vi "SequenceStructures.vi"() -> ()   [LabVIEW 2025]
uses:
  <vilib>/numeric/Random Number (Range) DBL.vi
panel:
  in  "Path 4":path
  out "Waveform Chart 4":dynamicdata(graph)
  in  "lower limit 2":dbl
  in  "upper limit 2":dbl
  in  "?":bool
  in  "write to file 2":bool
  in  "Path 3":path
  out "temperature 2":dbl
  out "Waveform Chart 3":dbl(graph)
  out "Waveform Chart 2":dynamicdata(graph)
  in  "Path 2":path
  in  "lower limit":dbl
  in  "upper limit":dbl
  in  "?":bool
  in  "write to file":bool
  in  "Path":path
  out "temperature":dbl
  out "Waveform Chart":dbl(graph)
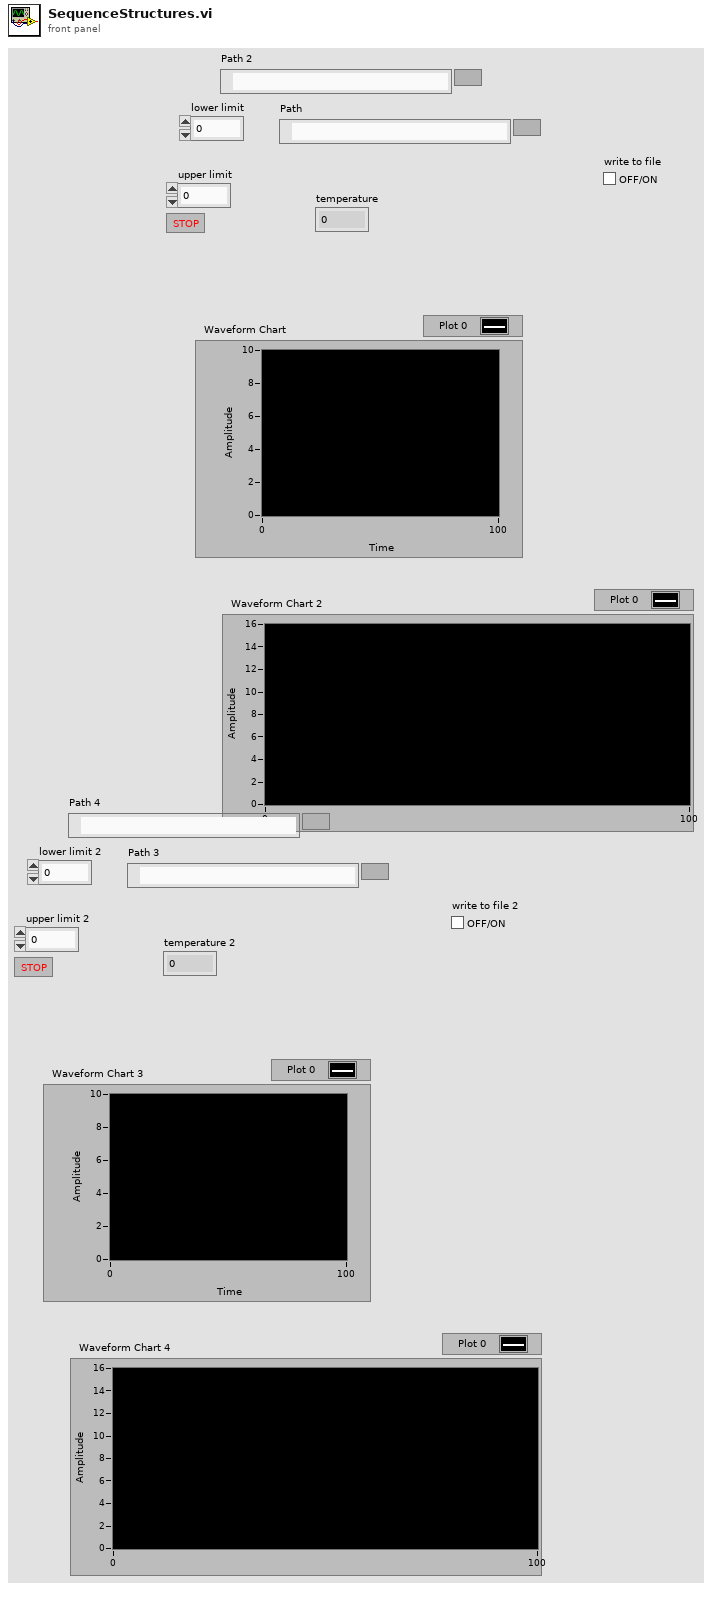
[diagram p1: front panel]
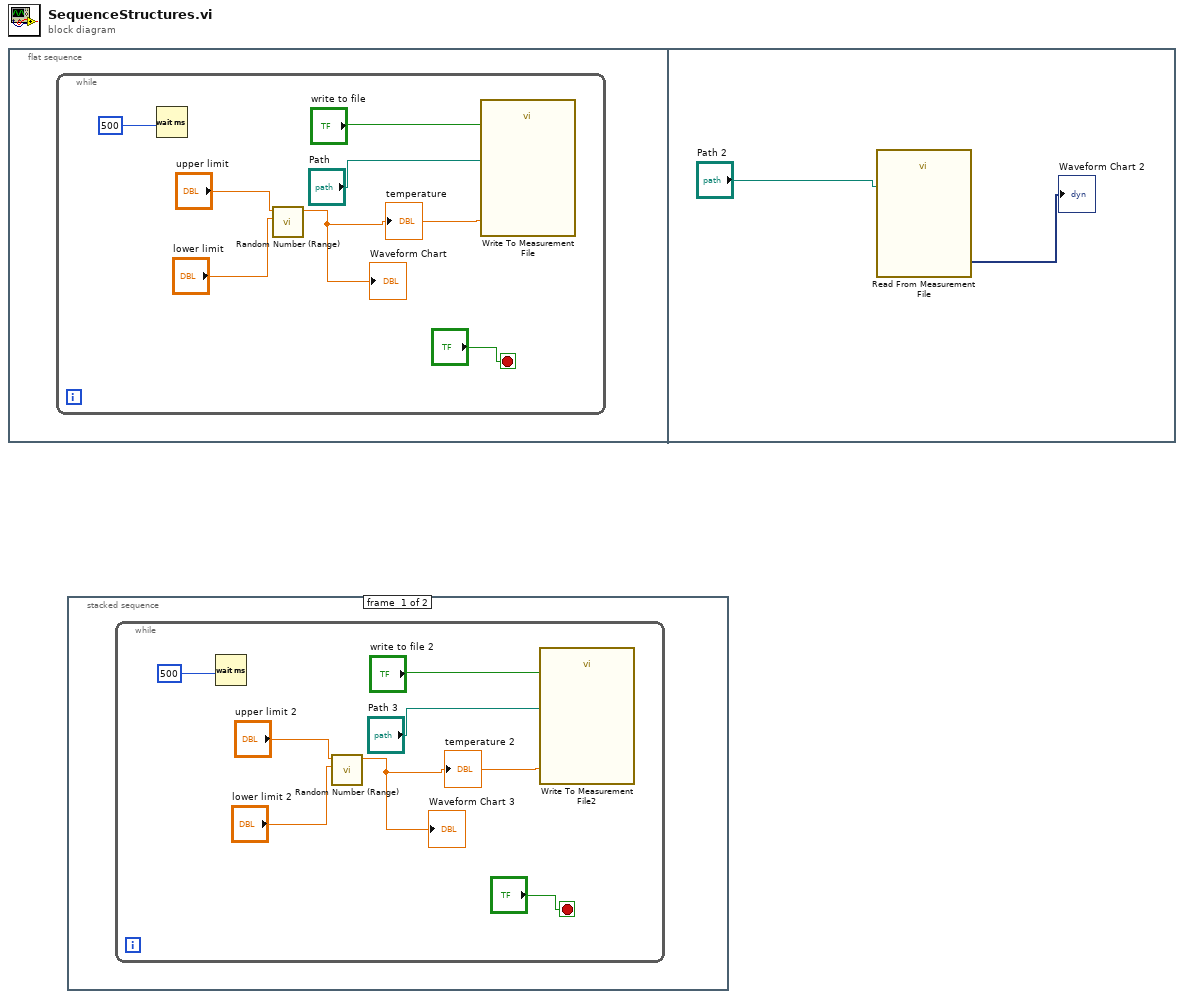
[diagram p0: block diagram]
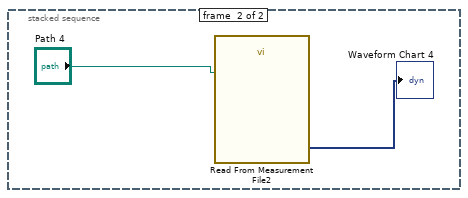
[diagram p2: hidden frame]
diagram:
  n1 = flat-sequence {
    frame #0 {
      n2 = while {
        stop <- "?" stop-if-true
        n3 = Wait (ms)(milliseconds to wait=u32 500 ("millisecond timer value")) -> ()  [unwired: 1 out]
        n4 = call-poly <vilib>:"Random Number (Range).vi"("lower bound (0)"="lower limit", "upper bound (100)"="upper limit") -> ("number"=w2:dbl)  [unwired: 9 in]
        "temperature" <- w2
        "Waveform Chart" <- w2
        n5 = call "Write To Measurement File"("Signals"=w2, "Enable"="write to file", "Filename"="Path") -> ()  [unwired: 14 in, 3 out]
      }
    }
    frame #1 {
      n6 = call "Read From Measurement File"("Filename"="Path 2") -> ("Signals"=→"Waveform Chart 2":dynamicdata)  [unwired: 5 in, 5 out]
    }
  }
  n7 = stacked-sequence {
    frame #0 {
      n8 = while {
        stop <- "?" stop-if-true
        n9 = Wait (ms)(milliseconds to wait=u32 500 ("millisecond timer value")) -> ()  [unwired: 1 out]
        n10 = call-poly <vilib>:"Random Number (Range).vi"("lower bound (0)"="lower limit 2", "upper bound (100)"="upper limit 2") -> ("number"=w11:dbl)  [unwired: 9 in]
        "temperature 2" <- w11
        "Waveform Chart 3" <- w11
        n11 = call "Write To Measurement File2"("Signals"=w11, "Enable"="write to file 2", "Filename"="Path 3") -> ()  [unwired: 14 in, 3 out]
      }
    }
    frame #1 {
      n12 = call "Read From Measurement File2"("Filename"="Path 4") -> ("Signals"=→"Waveform Chart 4":dynamicdata)  [unwired: 5 in, 5 out]
    }
  }
